vi "Rollover handler-Funct acq protocols.vi"(9 "Tick Count Register in":u32, 11 "Stimulus Trigger Setup":T1={"Trigger period in live protocols (80MHz Cycles)"=0, "Pulse width in live protocols (80MHz Cycles)"=0, "Enable stimulus in live protocols"=FALSE, "Trigger delay in funct. protocols (80MHz Cycles)"=400000, "Pulse width in funct. protocols (80MHz Cycles)"=400000, "Enable stimulus in funct. protocols"=FALSE}) -> (0 "Raw count":u32, 1 "Tick Count Register out":u32, 2 "Elapsed ticks count":u32, 3 "Target reached":bool)   [LabVIEW 2020]
uses:
  FPGA Typedefs/Stimulus trigger delays cluster.ctl
panel:
  # "Limited to 53.5 sec (if U32)"
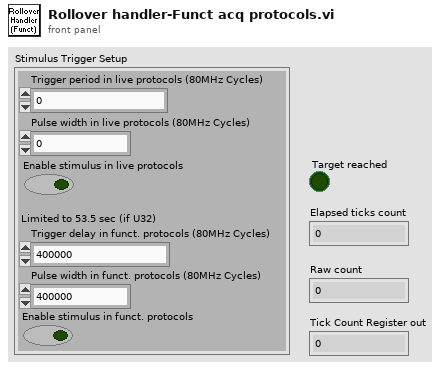
[diagram p1: front panel]
types:
  T1 = typedef "Stimulus trigger delays cluster.ctl" = cluster{"Trigger period in live protocols (80MHz Cycles)":u32, "Pulse width in live protocols (80MHz Cycles)":u32, "Enable stimulus in live protocols":bool, "Trigger delay in funct. protocols (80MHz Cycles)":u32, "Pulse width in funct. protocols (80MHz Cycles)":u32, "Enable stimulus in funct. protocols":bool}
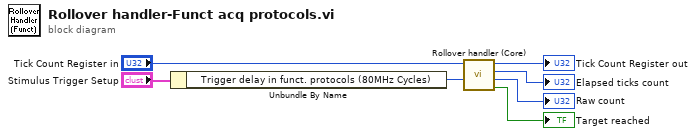
[diagram p0: block diagram]
diagram:
  n1 = Unbundle By Name("Stimulus Trigger Setup") -> ("Trigger delay in funct. protocols (80MHz Cycles)"=w1:u32)
  n2 = call "Rollover handler (Core).vi"("Target delay"=w1, "Tick Count Register in"="Tick Count Register in") -> ("Target delay reached"=→"Target reached":bool, "Raw count"=→"Raw count":u32, "Elapsed ticks count"=→"Elapsed ticks count":u32, "Tick Count Register out"=→"Tick Count Register out":u32)  [unwired: 6 in]
